vi "Go To Next Valid Step.vi"(8 "error in (no error)":errorcluster, 11 "Output Sequencer in":refnum<class "Output Sequencer.lvclass">) -> (0 "error out":errorcluster, 3 "Output Sequencer out":refnum<class "Output Sequencer.lvclass">, 5 "Sequencer State":T1)   [LabVIEW 2020, in "Output Sequencer.lvlib" / "Output Sequencer.lvclass"]
uses:
  Output Sequencer.lvclass
  Types/Sequencer State.ctl
  Output Sequencer.lvclass/Output Sequencer.ctl
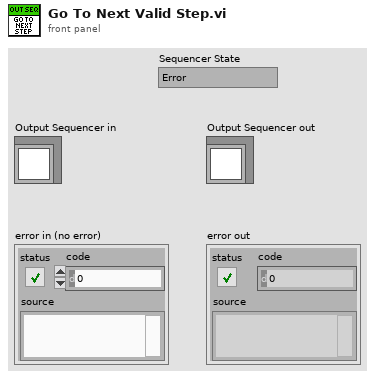
[diagram p1: front panel]
types:
  T1 = typedef "Output Sequencer.lvlib/Output Sequencer.lvclass/Sequencer State.ctl" = enum16{"Error", "Initialize", "Prepare channels", "Wait for test", "Wait for %.1f sec", "Wait for trigger", "Stop condition", "Wait for resume", "Running", "Paused", "No valid step", "Stopped"}
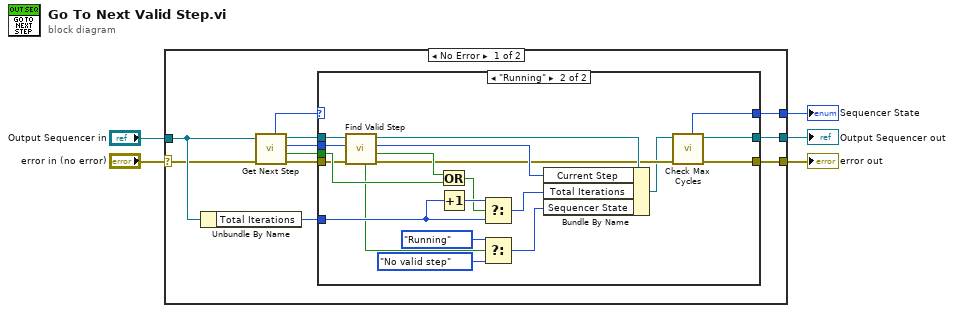
[diagram p0: block diagram]
diagram:
  n1 = case shown="No Error" "error in (no error)" {
    selector: "error in (no error)" -> [w6 w41]
    tunnel: [w16 w41] -> w5
    tunnel: [w15 w40] -> w4
    tunnel: "Output Sequencer in" -> [w14 w40]
    tunnel: [w7 _] -> w2
    frame No Error {
      n2 = Unbundle By Name(w14) -> ("Total Iterations"=w10:i32)
      n3 = call "Get Next Step.vi"("error in (no error)"=w6, "Output Sequencer in"=w14) -> ("error out"=w9:errorcluster, "Next Cycle?"=w12:bool, "Next Step"=w13:i32, "Output Sequencer out"=w11:refnum<class "Output Sequencer.lvclass">, "Sequencer State"=w8:T1)  [unwired: 5 in]
      n4 = case shown="\"Running\"" w8 {
        selector: w8 -> [w17 _]
        tunnel: [w18 w39] -> w16
        tunnel: [w19 w38] -> w15
        tunnel: w13 -> [_ w37]
        tunnel: w12 -> [_ w35]
        tunnel: w11 -> [w19 w34]
        tunnel: w10 -> [_ w31]
        tunnel: w9 -> [w18 w30]
        tunnel: [w17 w28] -> w7
        frame Default {
        }
        frame "Running" {
          n5 = call "Find Valid Step.vi"("error in (no error)"=w30, "Starting Step"=w37, "Output Sequencer in"=w34) -> ("error out"=w29:errorcluster, "Next Cycle?"=w36:bool, "Next Step"=w32:i32, "Output Sequencer out"=w33:refnum<class "Output Sequencer.lvclass">, "Valid Step Found"=w23:bool)  [unwired: 4 in]
          n6 = Or(x=w36, y=w35) -> (x .or. y?=w25:bool)
          n7 = Increment(x=w31) -> (x+1=w26:i32)
          n8 = Select(t=w26, s=w25, f=w31) -> (s? t:f=w24:i32)
          n9 = Select(t=Sequencer_State."Running" ("Sequencer State"), s=w23, f=Sequencer_State."No valid step" ("Sequencer State")) -> (s? t:f=w20:T1)
          n10 = Bundle By Name(cluster=w33, "Current Step"=w32, "Total Iterations"=w24, "Sequencer State"=w20) -> (w27:refnum<class "Output Sequencer.lvclass">)
          n11 = call "Check Max Cycles.vi"("error in (no error)"=w29, "Output Sequencer in"=w27) -> ("error out"=w39:errorcluster, "Output Sequencer out"=w38:refnum<class "Output Sequencer.lvclass">, "Sequencer State"=w28:T1)  [unwired: 6 in, 1 out]
        }
      }
    }
    frame Error {
    }
  }
  "error out" <- w5
  "Output Sequencer out" <- w4
  "Sequencer State" <- w2
